vi "process.vi"(8 "error in":errorcluster, 9 "result allocation":T1, 10 "parameters":T1, 11 "module in":refnum<class "user tag bus module.lvclass">) -> (0 "error out":errorcluster, 1 "results":T1, 2 "parameter allocation":T1, 3 "module out":refnum<class "user tag bus module.lvclass">)   [LabVIEW 2013, in "user tag bus module.lvclass"]
doc: "Provides an interface for information processing by a module at runtime. While this interface performs no operations, a child should provide an override which may process data in any manner necessary."
uses:
  user tag bus module.lvclass
  <vilib>/NI/Tag Bus/table/data table.ctl
  user tag bus module.lvclass/user tag bus module.ctl
  <vilib>/NI/Tag Bus/table/data table.lvlib
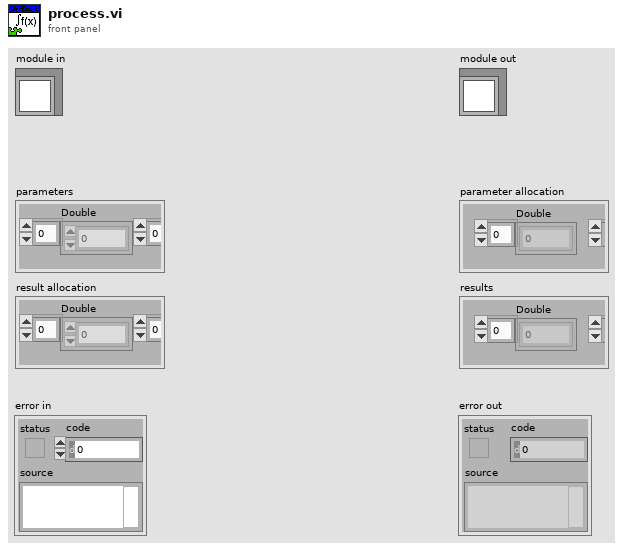
[diagram p1: front panel]
types:
  T1 = typedef "tag bus.lvlib/data table.lvlib/data table.ctl" = cluster{"Double":dbl[], "Single":sgl[], "I64":i64[], "I32":i32[], "I16":i16[], "I8":i8[], "U64":u64[], "U32":u32[], "U16":u16[], "U8":u8[], "Boolean":bool[], "String":string[], "Array of Double":cluster{"DBL Array":dbl[]}[], "Array of Single":cluster{"SGL Array":sgl[]}[], "Array of I64":cluster{"I64 Array":i64[]}[], "Array of I32":cluster{"I32 Array":i32[]}[], "Array of I16":cluster{"I16 Array":i16[]}[], "Array of I8":cluster{"I8 Array":i8[]}[], "Array of U64":cluster{"U64 Array":u64[]}[], "Array of U32":cluster{"U32 Array":u32[]}[], "Array of U16":cluster{"U16 Array":u16[]}[], "Array of U8":cluster{"U8 Array":u8[]}[], "Array of Boolean":cluster{"Boolean Array":bool[]}[], "Array of String":cluster{"String Array":string[]}[]}
  T2 = typedef "user tag bus module.lvclass/state control.ctl" = cluster{"control index (dbl)":i32, "output index (dbl)":i32}
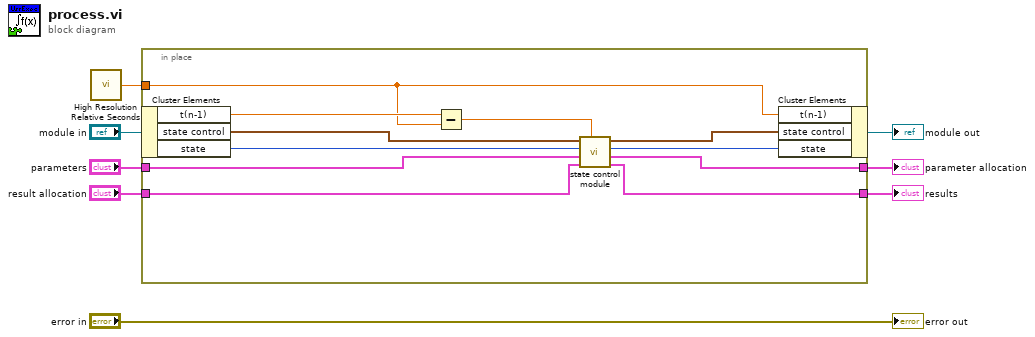
[diagram p0: block diagram]
diagram:
  n1 = call <vilib>:"High Resolution Relative Seconds.vi"() -> ("relative seconds"=w1:dbl)
  n2 = in-place {
    in-place-border: "parameters" -> [w11]
    in-place-border: "result allocation" -> [w12]
    in-place-border: [w14] -> w3
    in-place-border: [w13] -> w2
    in-place-border: w1 -> [w16]
    n3 = in-place-cluster #1("module in") -> ("t(n-1)"=w17:dbl, "state control"=w19:T2, "state"=w9:u8)
    n4 = Subtract(x=w17, y=w16) -> (x-y=w15:dbl)
    n5 = call "state control module.vi"("dt"=w15, "results in"=w12, "parameters in"=w11, "state in"=w9, "state control in"=w19) -> ("results out"=w14:T1, "parameters out"=w13:T1, "state out"=w10:u8, "state control out"=w18:T2)  [unwired: 3 in]
    n6 = in-place-cluster #1("t(n-1)"=w16, "state control"=w18, "state"=w10) -> (→"module out":refnum<class "user tag bus module.lvclass">)
  }
  "results" <- w3
  "parameter allocation" <- w2
  "error out" <- "error in"
